vi "Read XNET Settings.vi"(8 "error in (no error)":errorcluster, 11 "J1939 configuration in":refnum<class "J1939 configuration.lvclass">) -> (0 "error out":errorcluster, 2 "XNET Settings":T1={"Select Interface"="CAN2", "Node Address"=1, "Node Name"=1}, 3 "J1939 configuration out":refnum<class "J1939 configuration.lvclass">)   [LabVIEW 2014, in "J1939 configuration.lvclass"]
uses:
  J1939 configuration.lvclass
  XNET Settings.ctl
  J1939 configuration.lvclass/J1939 configuration.ctl
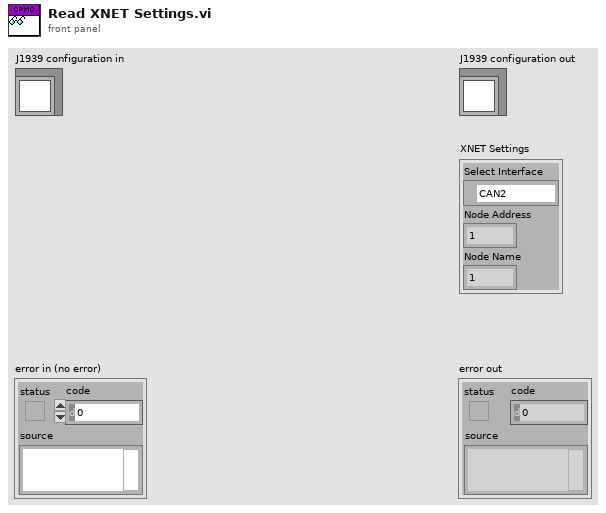
[diagram p1: front panel]
types:
  T1 = typedef "J1939 configuration.lvclass/XNET Settings.ctl" = cluster{"Select Interface":refnum<k21>, "Node Address":u8, "Node Name":u64}
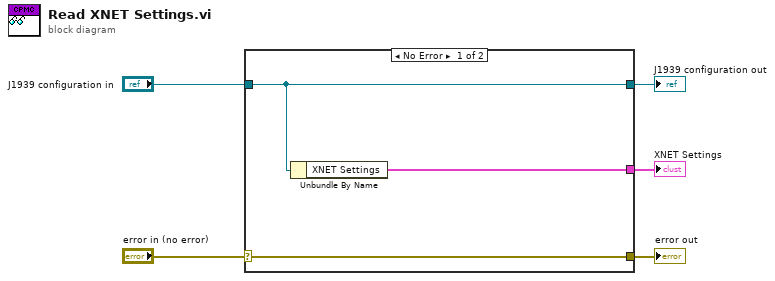
[diagram p0: block diagram]
diagram:
  n1 = case shown="No Error" "error in (no error)" {
    selector: "error in (no error)" -> [w8 w9]
    tunnel: [w8 w9] -> w4
    tunnel: [w7 w10] -> w2
    tunnel: "J1939 configuration in" -> [w7 w10]
    tunnel: [w6 _] -> w1
    frame No Error {
      n2 = Unbundle By Name(w7) -> ("XNET Settings"=w6:T1)
    }
    frame Error {
    }
  }
  "error out" <- w4
  "J1939 configuration out" <- w2
  "XNET Settings" <- w1
